vi "Main Page.vi"(8 "error in (no error)":errorcluster, 11 "Node Ptr":T5 format="%.0x") -> (0 "error out":errorcluster)   [LabVIEW 2015, in "Diagnostics Addon System Explorer.lvlib"]
uses:
  Diagnostics Addon System Explorer.lvlib
  <vilib>/NI Veristand/Custom Device API/Custom Device API.lvlib
  Shared/SubVIs/GUID Lookup.vi
  Shared/Diagnostics Addon Shared.lvlib
  <vilib>/NI Veristand/Custom Device API/Set Item Property (Variant).vi
  Types/FG.Action.ctl
  Types/Status.Export.ctl
  Types/Command.Export.ctl
  Shared/Types/986x.ctl
  Types/DTC.Export.ctl
  Shared/Types/DPID.Rate.ctl
  Shared/Types/DPID.ctl
  Types/DPID.Export.ctl
  Types/DPIDs.Export.ctl
  Shared/Types/Signal.ctl
  Types/Frame.Export.ctl
  Types/Frames.Export.ctl
  Shared/Types/Transport.ctl
  Shared/Types/Protocol.ctl
  Shared/Types/CAN.Interface.ctl
  Shared/Types/CAN.ctl
  Types/SysDef.Export.ctl
  Shared/Types/Security.ctl
  Types/CmdResp.Export.ctl
  Types/Routine.Export.ctl
  Types/Routines.Export.ctl
  Types/IO.Export.ctl
  Types/IOControls.Export.ctl
  <vilib>/NI Veristand/Custom Device API/Get Item Property (Boolean).vi
  Types/DTCControl.Export.ctl
  Shared/Types/DTCDescriptor.ctl
  <vilib>/NI Veristand/Custom Device API/Custom Device Item Ref.ctl
panel:
  in  "Tab Control":T1(tab)
  in  "Termination":bool
  in  "Name":string
  in  "Description":string
  out "Diagnostic Protocol":T2
  in  "CAN Interface":T3
  in  "Baud Rate":u32=250000
  in  "Enable Stream":bool
  in  "Fill Byte":u8=255 format="%.0x"
  in  "Fill Frame":bool
  in  "VW TP Channel ID":u32 format="%.0x"
  in  "Transport Protocol":T4
  in  "Receive UUDT ID":u32 format="%.0x"
  in  "Receive Extension":u8 format="%.0x"
  in  "Receive ID":u32 format="%.0x"
  in  "Transmit Extension":u8 format="%.0x"
  in  "Transmit ID":u32 format="%.0x"
  in  "Seed Key DLL Path":path
  in  "Enable Bitfile":bool
  in  "RIO Device":u16
  in  "Bitfile Path":path
  in  "Database File":path
  in  "Header":cluster{"Section Name":string}={"Section Name"="Custom Device Item Settings"}
  in  "SHDocVw.IWebBrowser":refnum<k7>(container)
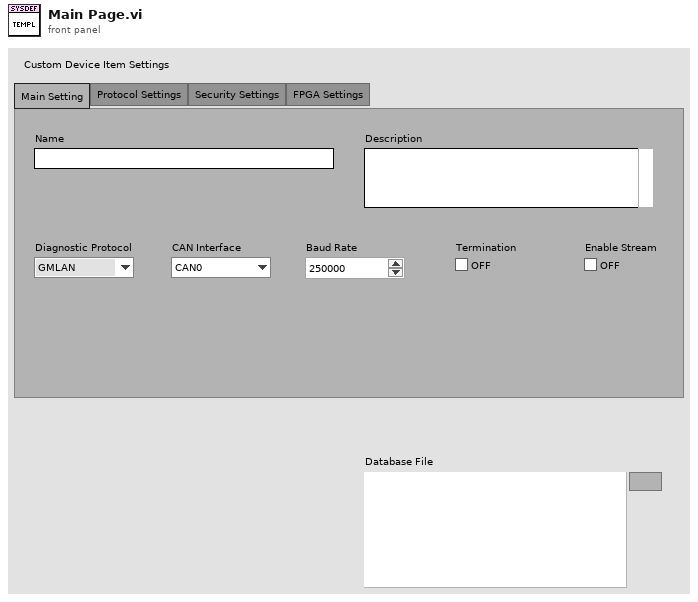
[diagram p1: front panel]
types:
  T1 = enum32{"Main Setting", "Protocol Settings", "Security Settings", "FPGA Settings"}
  T2 = typedef "Diagnostics Addon Shared.lvlib/Protocol.ctl" = enum16{"GMLAN", "KWP-2000", "UDS"}
  T3 = typedef "Diagnostics Addon Shared.lvlib/CAN.Interface.ctl" = enum16{"CAN0", "CAN1", "CAN2", "CAN3", "CAN4", "CAN5", "CAN6", "CAN7", "CAN8", "CAN9", "CAN10", "CAN11", "CAN12", "CAN13", "CAN14", "CAN15", "CAN16", "CAN17", "CAN18", "CAN19", "CAN20", "CAN21", "CAN22", "CAN23", "CAN24", "CAN25", "CAN26", "CAN27", "CAN28", "CAN29", "CAN30", "CAN31", "CAN32", "CAN33", "CAN34", "CAN35", "CAN36", "CAN37", "CAN38", "CAN39", "CAN40", "CAN41", "CAN42", "CAN43", "CAN44", "CAN45", "CAN46", "CAN47", "CAN48", "CAN49", "CAN50", "CAN51", "CAN52", "CAN53", "CAN54", "CAN55", "CAN56", "CAN57", "CAN58", "CAN59", "CAN60", "CAN61", "CAN62", "CAN63", "CAN 256 (Virtual)", "CAN 257 (Virtual)"}
  T4 = typedef "Diagnostics Addon Shared.lvlib/Transport.ctl" = enum16{"ISO TP - Normal Mode", "ISO TP - Mixed Mode", "VW TP 2.0", "Diagnostics on IP"}
  T5 = typedef "Custom Device API.lvlib/Custom Device Item Ref.ctl" = u64
  T6 = typedef "Diagnostics Addon System Explorer.lvlib/FG.Action.ctl" = enum16{"Get", "Set"}
  T7 = typedef "Custom Device API.lvlib/Custom Device Item Info.ctl" = cluster{"Name":string, "Is Channel":bool, "GUID":string, "Is Waveform":bool}
  T8 = typedef "Diagnostics Addon Shared.lvlib/CAN.ctl" = cluster{"CAN Interface":T3, "Baud Rate":u32, "Diagnostic Protocol":T2, "Transport Protocol":T4, "Transmit ID":u32, "Receive ID":u32, "Transmit Extension":u8, "Receive Extension":u8, "Receive UUDT ID":u32, "Enable Stream":bool, "VW TP Channel ID":u32, "Security":T9, "Fill Frame":bool, "Fill Byte":u8, "Termination":bool}
  T9 = typedef "Diagnostics Addon Shared.lvlib/Security.ctl" = cluster{"Source DLL Path":path, "Security Level":u8, "Target DLL Path":path}
  T10 = typedef "Diagnostics Addon System Explorer.lvlib/SysDef.Export.ctl" = cluster{"Name":string, "Description":string, "Diagnostics Basic Configuraiton":T11, "DID Outputs":T12, "DID Inputs":T12, "PID Outputs":T12, "PID Inputs":T12, "DPIDs":T15, "DTC":T19, "NI 986x Support":T22, "Commands":T23, "Status":T24, "IO Controls":T25, "Routines":T28, "Memory Outputs":T12, "Memory Inputs":T12}
  T11 = typedef "Diagnostics Addon Shared.lvlib/CAN.ctl" = cluster{"Database File":path, "CAN Interface":T3, "Baud Rate":u32, "Diagnostic Protocol":T2, "Transport Protocol":T4, "Transmit ID":u32, "Receive ID":u32, "Transmit Extension":u8, "Receive Extension":u8, "Receive UUDT ID":u32, "Enable Stream":bool, "VW TP Channel ID":u32, "Security":T9, "Fill Frame":bool, "Fill Byte":u8, "Termination":bool}
  T12 = typedef "Diagnostics Addon System Explorer.lvlib/Frames.Export.ctl" = cluster{"Description":string, "Frames":T13[]}
  T13 = typedef "Diagnostics Addon System Explorer.lvlib/Frame.Export.ctl" = cluster{"Name":string, "Description":string, "ID":u32, "Signals":T14[]}
  T14 = typedef "Diagnostics Addon Shared.lvlib/Signal.ctl" = cluster{"Start Bit":u8, "Length":u8, "Scaling Factor":dbl, "Scaling Offset":dbl, "Minimum":dbl, "Maximum":dbl, "Data Type":u32, "Byte Order":u32, "Default Value":dbl, "Name":string, "Units":string, "Description":string}
  T15 = typedef "Diagnostics Addon System Explorer.lvlib/DPIDs.Export.ctl" = cluster{"Description":string, "DPIDs":T16[]}
  T16 = typedef "Diagnostics Addon System Explorer.lvlib/DPID.Export.ctl" = cluster{"Name":string, "Description":string, "DPID":T17}
  T17 = typedef "Diagnostics Addon Shared.lvlib/DPID.ctl" = cluster{"DPID ID":u8, "Speed":T18, "PIDs":u16[]}
  T18 = typedef "Diagnostics Addon Shared.lvlib/DPID.Rate.ctl" = enum16{"Slow", "Medium", "Fast"}
  T19 = typedef "Diagnostics Addon System Explorer.lvlib/DTC.Export.ctl" = cluster{"Description":string, "DTC descriptor":T20, "DTC Control":T21}
  T20 = typedef "Diagnostics Addon Shared.lvlib/DTCDescriptor.ctl" = cluster{"DTC Byte Length":i32, "Status Byte Length":i32, "Add Data Byte Length":i32, "Byte Order":enum16{"Motorola", "Intel"}}
  T21 = typedef "Diagnostics Addon System Explorer.lvlib/DTCControl.Export.ctl" = cluster{"Description":string, "Signals":T14[]}
  T22 = typedef "Diagnostics Addon Shared.lvlib/986x.ctl" = cluster{"Enable 986x":bool, "RIO Device":u16, "Bitfile":path}
  T23 = typedef "Diagnostics Addon System Explorer.lvlib/Command.Export.ctl" = cluster{"Description":string}
  T24 = typedef "Diagnostics Addon System Explorer.lvlib/Status.Export.ctl" = cluster{"Description":string}
  T25 = typedef "Diagnostics Addon System Explorer.lvlib/IOControls.Export.ctl" = cluster{"Description":string, "IO Control Array":T26[]}
  T26 = typedef "Diagnostics Addon System Explorer.lvlib/IO.Export.ctl" = cluster{"Name":string, "Description":string, "ID":u16, "Signals":T27}
  T27 = typedef "Diagnostics Addon System Explorer.lvlib/CmdResp.Export.ctl" = cluster{"Cmd":T14[], "Response":T14[]}
  T28 = typedef "Diagnostics Addon System Explorer.lvlib/Routines.Export.ctl" = cluster{"Description":string, "Routine Array":T29[]}
  T29 = typedef "Diagnostics Addon System Explorer.lvlib/Routine.Export.ctl" = cluster{"Name":string, "Description":string, "ID":u16, "Start Parameters":T27, "Request Parameters":T27, "Stop Parameters":T27}
  T30 = typedef "Custom Device API.lvlib/Custom Device Commands.ctl" = enum16{"Default", "Item renamed", "Shutdown", "Dynamic button pressed"}
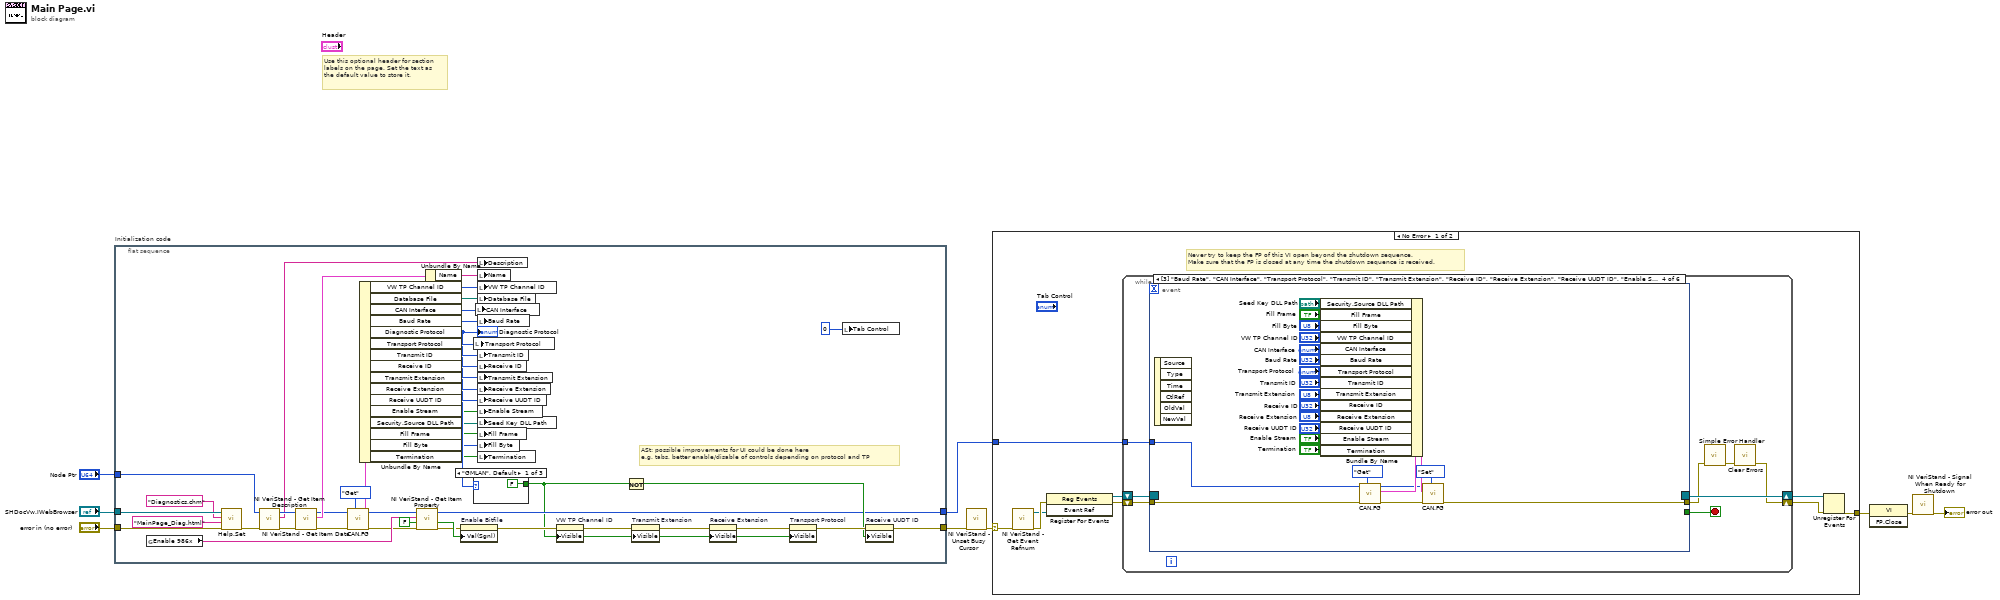
[diagram p0: block diagram]
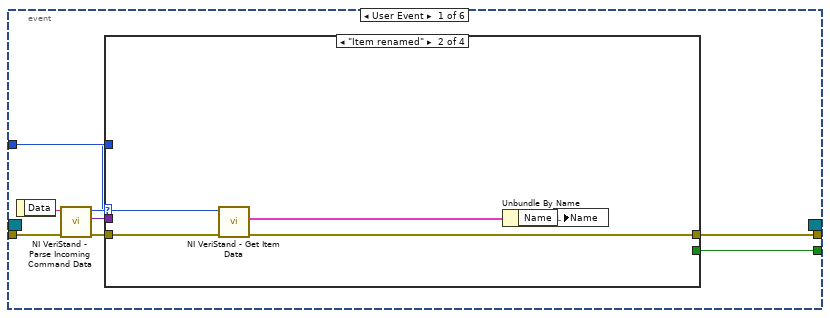
[diagram p2: hidden frame]
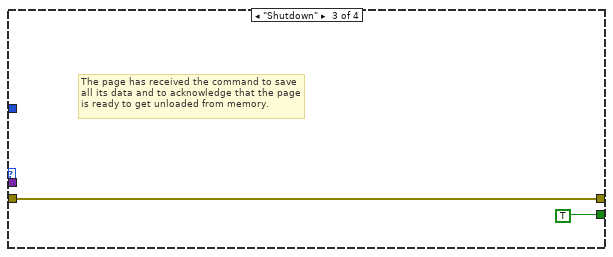
[diagram p4: hidden frame]
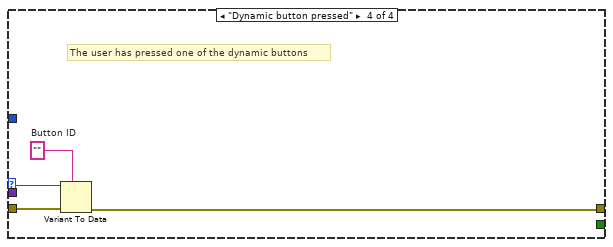
[diagram p5: hidden frame]
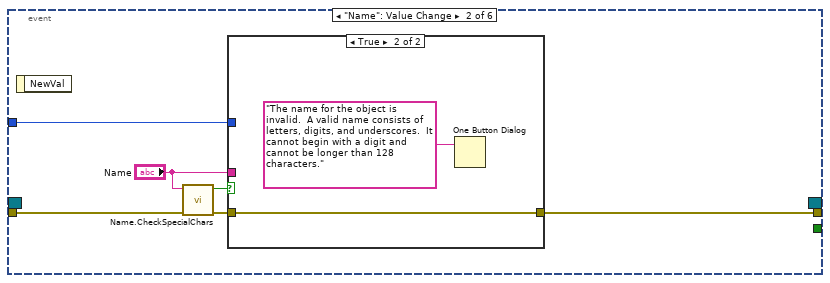
[diagram p6: hidden frame]
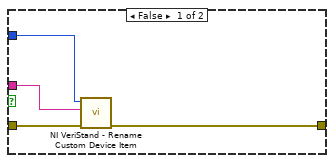
[diagram p7: hidden frame]
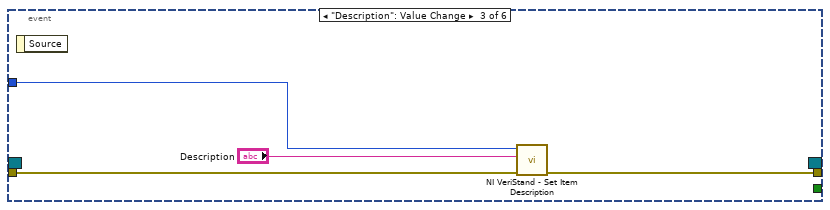
[diagram p8: hidden frame]
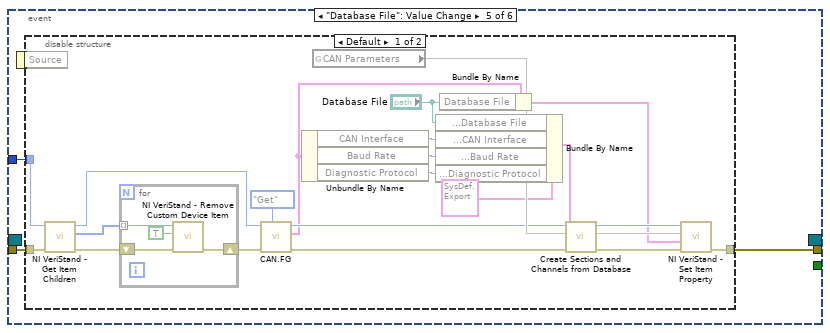
[diagram p9: hidden frame]
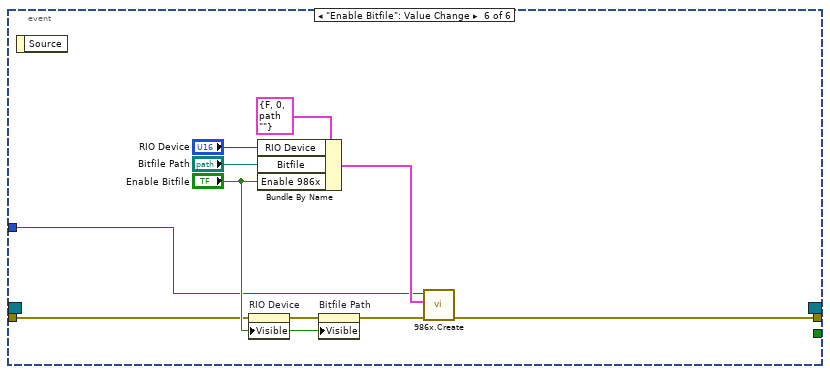
[diagram p11: hidden frame]
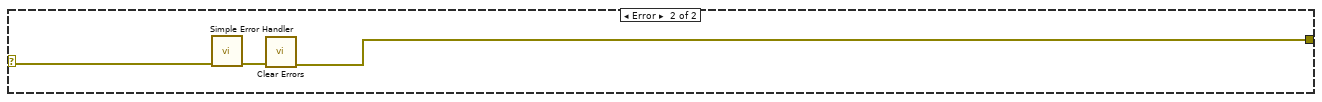
[diagram p12: hidden frame]
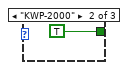
[diagram p13: hidden frame]
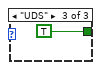
[diagram p14: hidden frame]
diagram:
  # "Use this optional header for section labels on the page. Set the text as the default value to store it."
  n1 = flat-sequence "Initialization code" {
    tunnel: "error in (no error)" -> [w50]
    tunnel: "Node Ptr" -> [w55]
    tunnel: [w21] -> w5
    tunnel: [w23] -> w2
    tunnel: "SHDocVw.IWebBrowser" -> [w48]
    frame #0 {
      # "ASt: possible improvements for UI could be done here\ne.g. tabs, better enable/disable of controls depending on protocol and TP"
      n2 = global read "GUID Lookup.vi" "Enable 986x"() -> (w28:string)
      n3 = call "Help.Set.vi"("error in (no error)"=w50, "HTML File"="MainPage_Diag.html", "Main CHM File"="Diagnostics.chm", "SHDocVw.IWebBrowser2"=w48) -> ("error out"=w49:errorcluster)  [unwired: 7 in]
      n4 = call <vilib>:"NI VeriStand - Get Item Description.vi"("error in (no error)"=w49, "Item Ref in"=w55) -> ("error out"=w53:errorcluster, "Description"=w54:string, "Item Ref out"=w56:T5)  [unwired: 7 out]
      n5 = call <vilib>:"NI VeriStand - Get Item Data.vi"("error in (no error)"=w53, "Item Ref in"=w56) -> ("error out"=w44:errorcluster, "Item Info"=w52:T7, "Item Ref out"=w45:T5)  [unwired: 7 out]
      n6 = call "CAN.FG.vi"("Action"=FG.Action."Get", "error in (no error)"=w44, "Device Item Ref in"=w45) -> ("error out"=w22:errorcluster, "Diagnostics Basic Configuraiton"=w43:T8, "Device Item Ref out"=w24:T5)  [unwired: 6 in]
      n7 = Unbundle By Name(w43) -> ("VW TP Channel ID"=w19:u32, "Database File"=w42:path, "CAN Interface"=w41:T3, "Baud Rate"=w40:u32, "Diagnostic Protocol"=w33:T2, "Transport Protocol"=w39:T4, "Transmit ID"=w38:u32, "Receive ID"=w37:u32, "Transmit Extension"=w36:u8, "Receive Extension"=w34:u8, "Receive UUDT ID"=w35:u32, "Enable Stream"=w20:bool, "Security.Source DLL Path"=w11:path, "Fill Frame"=w12:bool, "Fill Byte"=w13:u8, "Termination"=w10:bool)
      "Diagnostic Protocol" <- w33
      n8 = call-poly <vilib>:"NI VeriStand - Get Item Property.vi"("error in (no error)"=w22, "Default Value"=FALSE, "Property Name"=w28, "Item Ref in"=w24) -> ("error out"=w25:errorcluster, "Value"=w26:bool, "Item Ref out"=w23:T5)  [unwired: 4 in, 1 out]
      n9 = Unbundle By Name(w52) -> ("Name"=w51:string)
      n10 = property on="Enable Bitfile" class="Bool (strict)"(error in=w25, "Val(Sgnl)"=w26) -> (error out=w17:errorcluster)  [unwired: 1 in, 1 out]
      n11 = local write "Transport Protocol"(w39) -> ()
      n12 = case shown="\"GMLAN\", Default" w33 {
        tunnel: [FALSE TRUE TRUE] -> w15
        frame "GMLAN", Default {
        }
        frame "KWP-2000" {
        }
        frame "UDS" {
        }
      }
      n13 = local write "CAN Interface"(w41) -> ()
      n14 = local write "Description"(w54) -> ()
      n15 = local write "Name"(w51) -> ()
      n16 = local write "VW TP Channel ID"(w19) -> ()
      n17 = local write "Database File"(w42) -> ()
      n18 = local write "Baud Rate"(w40) -> ()
      n19 = local write "Transmit ID"(w38) -> ()
      n20 = local write "Receive ID"(w37) -> ()
      n21 = local write "Transmit Extension"(w36) -> ()
      n22 = local write "Receive Extension"(w34) -> ()
      n23 = local write "Receive UUDT ID"(w35) -> ()
      n24 = local write "Enable Stream"(w20) -> ()
      n25 = local write "Seed Key DLL Path"(w11) -> ()
      n26 = local write "Fill Frame"(w12) -> ()
      n27 = local write "Fill Byte"(w13) -> ()
      n28 = local write "Termination"(w10) -> ()
      n29 = property on="VW TP Channel ID" class="DigNum (strict)"(error in=w17, "Visible"=w15) -> (error out=w16:errorcluster)  [unwired: 1 in, 1 out]
      n30 = Not(x=w15) -> (.not. x?=w29:bool)
      n31 = property on="Transmit Extension" class="DigNum (strict)"(error in=w16, "Visible"=w15) -> (error out=w32:errorcluster)  [unwired: 1 in, 1 out]
      n32 = property on="Receive Extension" class="DigNum (strict)"(error in=w32, "Visible"=w15) -> (error out=w31:errorcluster)  [unwired: 1 in, 1 out]
      n33 = property on="Transport Protocol" class="Enum (strict)"(error in=w31, "Visible"=w15) -> (error out=w30:errorcluster)  [unwired: 1 in, 1 out]
      n34 = local write "Tab Control"(0) -> ()
      n35 = property on="Receive UUDT ID" class="DigNum (strict)"(error in=w30, "Visible"=w29) -> (error out=w21:errorcluster)  [unwired: 1 in, 1 out]
    }
  }
  n36 = call <vilib>:"NI VeriStand - Unset Busy Cursor.vi"("error in (no error)"=w5) -> ("error out"=w4:errorcluster)  [unwired: 10 out]
  n37 = case shown="No Error" w4 {
    selector: w4 -> [w60 w177]
    tunnel: [w65 w175] -> w9
    tunnel: w2 -> [w61 _]
    frame No Error {
      # "Never try to keep the FP of this VI open beyond the shutdown sequence.\nMake sure that the FP is closed at any time the shutdown sequence is received."
      n38 = call <vilib>:"NI VeriStand - Get Event Refnum.vi"("error in (no error)"=w60) -> ("error out"=w68:errorcluster, "Event Ref"=w64:refnum<user-event>)  [unwired: 9 out]
      n39 = register-events(error in=w68, w64) -> (reference out=w62:refnum<event-registration>, error out=w63:errorcluster)  [unwired: 1 in]
      n40 = while {
        tunnel: w61 -> [w72]
        shift-right: [w69] -> w66
        shift-left: w63 -> [w75]
        shift-right: [w76] -> w67
        shift-left: w62 -> [w74]
        stop <- w73 stop-if-true
        n41 = event shown="[3] \"Baud Rate\", \"CAN Interface\", \"Transport Protocol\", \"Transmit ID\", \"Transmit Extension\", \"Receive ID\", \"Receive Extension\", \"Receive UUDT ID\", \"Enable Stream\", \"VW TP Channel ID\", \"Fill Frame\", \"Fill Byte\", \"Termination\": Value Change" {
          selector: w74 -> [_ _ _ _ _ _]
          dyn-events: [_ _ _ _ _ _] -> w76
          timeout: _ -> [_ _ _ _ _ _]
          tunnel: w75 -> [w84 w99 w111 w135 w137 w168]
          tunnel: [w80 _ _ _ _ _] -> w73
          tunnel: [w79 w102 w110 w118 w138 w166] -> w71
          tunnel: w72 -> [w78 w101 w112 w134 w136 w165]
          event User Event {
            n42 = event-data() -> ("Data"=w83:string)  [unwired: 1 out]
            n43 = call <vilib>:"NI VeriStand - Parse Incoming Command Data.vi"("error in (no error)"=w84, "Incoming data"=w83) -> ("error out"=w82:errorcluster, "Outgoing data"=w77:variant, "Action"=w81:T30)  [unwired: 7 out]
            n44 = case shown="\"Item renamed\"" w81 {
              tunnel: w82 -> [w85 w90 w91 w96]
              tunnel: [_ _ TRUE _] -> w80
              tunnel: [w85 w87 w91 w93] -> w79
              tunnel: w78 -> [_ w89 _ _]
              tunnel: w77 -> [_ _ _ w95]
              frame "Default", Default {
              }
              frame "Item renamed" {
                n45 = call <vilib>:"NI VeriStand - Get Item Data.vi"("error in (no error)"=w90, "Item Ref in"=w89) -> ("error out"=w87:errorcluster, "Item Info"=w88:T7)  [unwired: 8 out]
                n46 = Unbundle By Name(w88) -> ("Name"=w86:string)
                n47 = local write "Name"(w86) -> ()
              }
              frame "Shutdown" {
                # "The page has received the command to save all its data and to acknowledge that the page is ready to get unloaded from memory."
              }
              frame "Dynamic button pressed" {
                w94 = ""  # Button ID
                # "The user has pressed one of the dynamic buttons"
                n48 = Variant To Data(error in=w96, type=w94, Variant=w95) -> (error out=w93:errorcluster)  [unwired: 1 out]
              }
            }
          }
          event "Name": Value Change {
            n49 = event-data() -> ()  [unwired: 2 out]
            n50 = call "Name.CheckSpecialChars.vi"("error in"=w99, "Signal Name"="Name") -> ("error out"=w98:errorcluster, "Special Character?"=w97:bool)  [unwired: 8 in]
            n51 = case shown="True" w97 {
              tunnel: [w106 w108] -> w102
              tunnel: w101 -> [w105 _]
              tunnel: "Name" -> [w104 _]
              tunnel: w98 -> [w103 w108]
              frame False {
                n52 = call <vilib>:"NI VeriStand - Rename Custom Device Item.vi"("error in (no error)"=w103, "New Name"=w104, "Item Ref in"=w105) -> ("error out"=w106:errorcluster)  [unwired: 1 in, 7 out]
              }
              frame True {
                n53 = One Button Dialog(message="The name for the object is invalid.  A valid name consists of letters, digits, and underscores.  It cannot begin with a digit and cannot be longer than 128 characters.") -> ()  [unwired: 1 in, 1 out]
              }
            }
          }
          event "Description": Value Change {
            n54 = event-data() -> ()  [unwired: 2 out]
            n55 = call <vilib>:"NI VeriStand - Set Item Description.vi"("error in (no error)"=w111, "Description"="Description", "Item Ref in"=w112) -> ("error out"=w110:errorcluster)  [unwired: 8 out]
          }
          event "Baud Rate", "Transmit ID", "Transmit Extension", "Receive ID", "Receive Extension", "Receive UUDT ID", "Enable Stream", "VW TP Channel ID", "Fill Frame", "Fill Byte", "Termination": Value Change {
            n56 = event-data() -> ()  [unwired: 7 out]
            n57 = call "CAN.FG.vi"("Action"=FG.Action."Get", "error in (no error)"=w135, "Device Item Ref in"=w134) -> ("error out"=w120:errorcluster, "Diagnostics Basic Configuraiton"=w133:T8, "Device Item Ref out"=w119:T5)  [unwired: 6 in]
            n58 = Bundle By Name(cluster=w133, "Security.Source DLL Path"="Seed Key DLL Path", "Fill Frame"="Fill Frame", "Fill Byte"="Fill Byte", "VW TP Channel ID"="VW TP Channel ID", "CAN Interface"="CAN Interface", "Baud Rate"="Baud Rate", "Transport Protocol"="Transport Protocol", "Transmit ID"="Transmit ID", "Transmit Extension"="Transmit Extension", "Receive ID"="Receive ID", "Receive Extension"="Receive Extension", "Receive UUDT ID"="Receive UUDT ID", "Enable Stream"="Enable Stream", "Termination"="Termination") -> (w121:T8)
            n59 = call "CAN.FG.vi"("Action"=FG.Action."Set", "error in (no error)"=w120, "Diagnostics Basic Configuraiton"=w121, "Device Item Ref in"=w119) -> ("error out"=w118:errorcluster)  [unwired: 5 in, 2 out]
          }
          event "Database File": Value Change {
            n60 = event-data() -> ()  [unwired: 2 out]
            n61 = disable-structure shown="Default" {
              disable-tunnel: [w158 w164] -> w138
              disable-tunnel: w137 -> [w157 w164]
              disable-tunnel: w136 -> [w156 _]
              frame condition #0 {
                n62 = call <vilib>:"NI VeriStand - Get Item Children.vi"("error in (no error)"=w157, "Item Ref in"=w156) -> ("error out"=w155:errorcluster, "Child Refs"=w154:T5[], "Item Ref out"=w152:T5)  [unwired: 6 in, 1 out]
                n63 = for {
                  shift-right: [w162] -> w153
                  shift-left: w155 -> [w163]
                  tunnel: w154 -> [w161] mode=indexing
                  n64 = call <vilib>:"NI VeriStand - Remove Custom Device Item.vi"("error in (no error)"=w163, "Force Delete (F)"=TRUE, "Item Ref in"=w161) -> ("error out"=w162:errorcluster)  [unwired: 7 in, 1 out]
                }
                n65 = call "CAN.FG.vi"("Action"=FG.Action."Get", "error in (no error)"=w153, "Device Item Ref in"=w152) -> ("error out"=w145:errorcluster, "Diagnostics Basic Configuraiton"=w143:T8, "Device Item Ref out"=w147:T5)  [unwired: 6 in]
                n66 = Unbundle By Name(w143) -> ("CAN Interface"=w151:T3, "Baud Rate"=w150:u32, "Diagnostic Protocol"=w149:T2)
                n67 = global read "GUID Lookup.vi" "CAN Parameters"() -> (w159)
                n68 = Bundle By Name(cluster=T10 {"Name"="", "Description"="", "Diagnostics Basic Configuraiton"={"Database File"=path "", "CAN Interface"=enum."CAN0", "Baud Rate"=0, "Diagnostic Protocol"=enum."GMLAN", "Transport Protocol"=enum."ISO TP - Normal Mode", "Transmit ID"=0, "Receive ID"=0, "Transmit Extension"=0, "Receive Extension"=0, "Receive UUDT ID"=0, "Enable Stream"=FALSE, "VW TP Channel ID"=0, "Security"={"Source DLL Path"=path "", "Security Level"=1, "Target DLL Path"=path ""}, "Fill Frame"=FALSE, "Fill Byte"=255, "Termination"=FALSE}, "DID Outputs"={"Description"="", "Frames"=[]}, "DID Inputs"={"Description"="", "Frames"=[]}, "PID Outputs"={"Description"="", "Frames"=[]}, "PID Inputs"={"Description"="", "Frames"=[]}, "DPIDs"={"Description"="", "DPIDs"=[]}, "DTC"={"Description"="", "DTC descriptor"={"DTC Byte Length"=0, "Status Byte Length"=0, "Add Data Byte Length"=0, "Byte Order"=enum."Motorola"}, "DTC Control"={"Description"="", "Signals"=[]}}, "NI 986x Support"={"Enable 986x"=FALSE, "RIO Device"=0, "Bitfile"=path ""}, "Commands"={"Description"=""}, "Status"={"Description"=""}, "IO Controls"={"Description"="", "IO Control Array"=[]}, "Routines"={"Description"="", "Routine Array"=[]}, "Memory Outputs"={"Description"="", "Frames"=[]}, "Memory Inputs"={"Description"="", "Frames"=[]}} ("Configuration"), "Diagnostics Basic Configuraiton.Database File"="Database File", "Diagnostics Basic Configuraiton.CAN Interface"=w151, "Diagnostics Basic Configuraiton.Baud Rate"=w150, "Diagnostics Basic Configuraiton.Diagnostic Protocol"=w149) -> (w141:T10)
                n69 = Bundle By Name(cluster=w143, "Database File"="Database File") -> (w142:T8)
                n70 = call "Create Sections and Channels from Database.vi"("error in (no error)"=w145, "Configuration"=w141, "Device Item Ref out in"=w147) -> ("error out"=w144:errorcluster, "Device Item Ref out out"=w146:T5)  [unwired: 7 in]
                n71 = call-poly <vilib>:"NI VeriStand - Set Item Property.vi"("error in (no error)"=w144, "Value"=w142, "Property Name"=w159, "Item Ref in"=w146) -> ("error out"=w158:errorcluster)  [unwired: 5 in, 2 out]
              }
              frame condition #1 (active) {
              }
            }
          }
          event "Enable Bitfile": Value Change {
            n72 = event-data() -> ()  [unwired: 2 out]
            n73 = property on="RIO Device" class="DigNum (strict)"(error in=w168, "Visible"="Enable Bitfile") -> (error out=w174:errorcluster)  [unwired: 1 in, 1 out]
            n74 = Bundle By Name(cluster=T22 {"Enable 986x"=FALSE, "RIO Device"=0, "Bitfile"=path ""} ("986x Support"), "RIO Device"="RIO Device", "Bitfile"="Bitfile Path", "Enable 986x"="Enable Bitfile") -> (w169:T22)
            n75 = property on="Bitfile Path" class="Path"(error in=w174, "Visible"="Enable Bitfile") -> (error out=w167:errorcluster)  [unwired: 1 in, 1 out]
            n76 = call "986x.Create.vi"("error in (no error)"=w167, "986x Support"=w169, "Device Item Ref in"=w165) -> ("error out"=w166:errorcluster)  [unwired: 7 in, 1 out]
          }
        }
        n77 = call <vilib>:"Simple Error Handler.vi"("error in (no error)"=w71) -> ("error out"=w70:errorcluster)  [unwired: 1 in, 7 out]
        n78 = call <vilib>:"Clear Errors.vi"("error in (no error)"=w70) -> ("error out"=w69:errorcluster)  [unwired: 1 in, 5 out]
      }
      n79 = Unregister For Events(event registration refnum=w67, error in=w66) -> (error out=w65:errorcluster)
    }
    frame Error {
      n80 = call <vilib>:"Simple Error Handler.vi"("error in (no error)"=w177) -> ("error out"=w176:errorcluster)  [unwired: 1 in, 7 out]
      n81 = call <vilib>:"Clear Errors.vi"("error in (no error)"=w176) -> ("error out"=w175:errorcluster)  [unwired: 1 in, 5 out]
    }
  }
  n82 = invoke class="VI" method="FP.Close"(error in=w9) -> (error out=w8:errorcluster)  [unwired: 2 in, 2 out]
  n83 = call <vilib>:"NI VeriStand - Signal When Ready for Shutdown.vi"("error in (no error)"=w8) -> ("error out"=→"error out":errorcluster)  [unwired: 10 out]
